vi "zadanie3.vi"() -> ()   [LabVIEW 2012]
panel:
  out "Lsowe liczby z zakresu <1,49>":dbl[](array[numeric])
  out "Nazwa użytkownika:":string
  # "Program losuje 6 liczb z zakresu <1,49>"
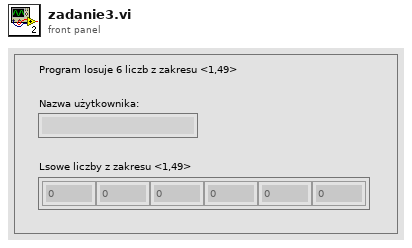
[diagram p1: front panel]
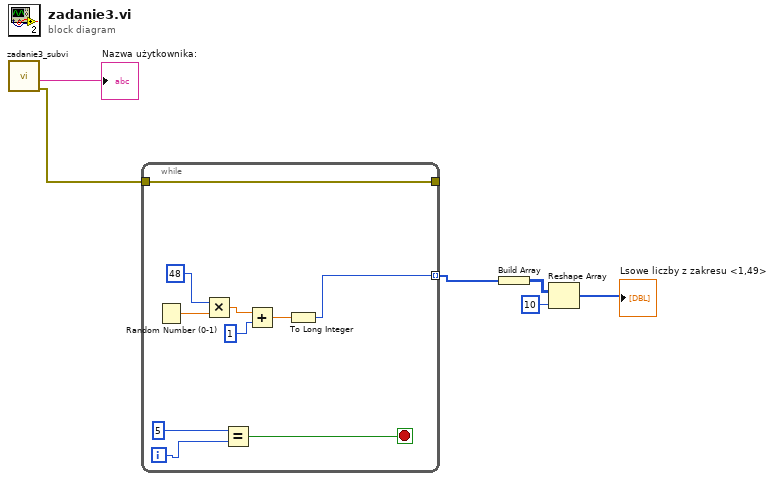
[diagram p0: block diagram]
diagram:
  n1 = call "zadanie3_subvi.vi"() -> ("error out"=w5:errorcluster, "Podaj login: out"=→"Nazwa użytkownika:":string)  [unwired: 7 in, 3 out]
  n2 = while {
    tunnel: w5 -> [w16]
    tunnel: [w16] -> _
    tunnel: [w7] -> w1 mode=indexing
    i -> [w14]
    stop <- w13 stop-if-true
    n3 = Random Number (0-1)() -> (number: 0 to 1=w11:dbl)
    n4 = Multiply(x=48, y=w11) -> (x*y=w10:dbl)
    n5 = Equal?(x=5, y=w14) -> (x = y?=w13:bool)
    n6 = Add(x=w10, y=1) -> (x+y=w8:dbl)
    n7 = To Long Integer(number=w8) -> (32bit integer=w7:i32)
  }
  n8 = Build Array(w1) -> (w3:i32[][])
  n9 = Reshape Array(w3, 10 ("dimension size")) -> (→"Lsowe liczby z zakresu <1,49>":i32[])
